vi "getMessage.vi"(8 "error in (no error)":errorcluster, 11 "SpectrographClientCommunicator in":refnum<class "SpectrographClientCommunicator.lvclass">) -> (0 "error out":errorcluster, 2 "message":string, 3 "SpectrographClientCommunicator out":refnum<class "SpectrographClientCommunicator.lvclass">)   [LabVIEW 2016, in "SpectrographClientCommunicator.lvclass"]
uses:
  SpectrographClientCommunicator.lvclass
  ts_labview_tcp/TCPClient/TCPClient.lvclass
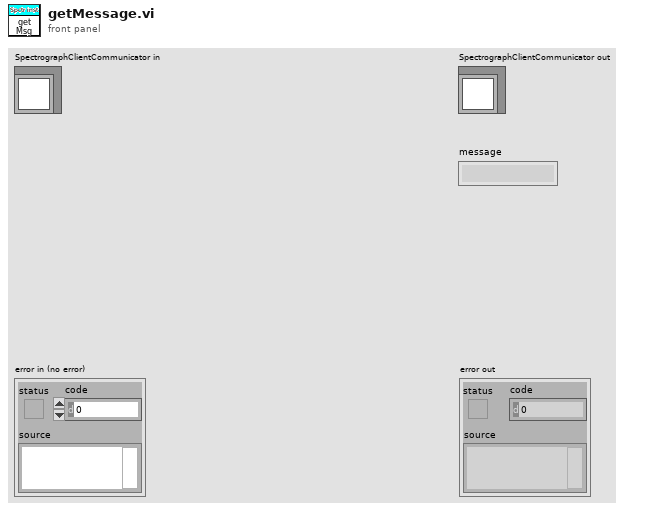
[diagram p1: front panel]
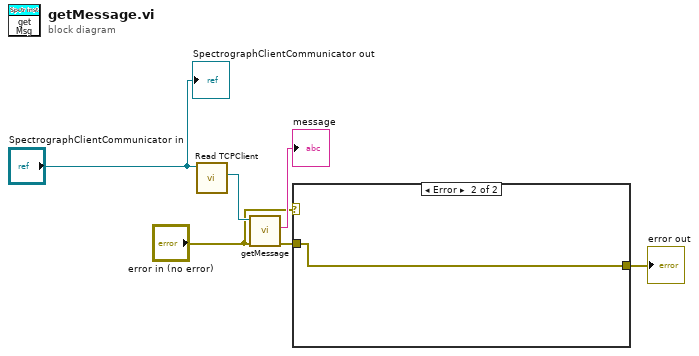
[diagram p0: block diagram]
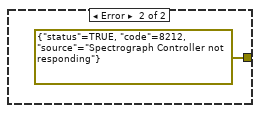
[diagram p3: hidden frame]
diagram:
  n1 = call-dynamic "Read TCPClient.vi"("SpectrographClientCommunicator in"="SpectrographClientCommunicator in") -> ("TCPClient"=w5:refnum<class "TCPClient.lvclass">)  [unwired: 8 in, 2 out]
  n2 = call-dynamic "getMessage.vi"("error in (no error)"="error in (no error)", "TCPClient in"=w5) -> ("error out"=w3:errorcluster, "String"=→"message":string)  [unwired: 7 in, 1 out]
  n3 = case shown="Error" "error in (no error)" {
    tunnel: w3 -> [w8 w11]
    tunnel: [w7 w11] -> w1
    frame No Error {
      n4 = case shown="No Error" w8 {
        selector: w8 -> [w9 _]
        tunnel: [w9 errorcluster {"status"=TRUE, "code"=8212, "source"="Spectrograph Controller not responding"} ("error IO")] -> w7
        frame No Error {
        }
        frame Error {
        }
      }
    }
    frame Error {
    }
  }
  "error out" <- w1
  "SpectrographClientCommunicator out" <- "SpectrographClientCommunicator in"
